vi "Send_string_to_MCU.vi"() -> (0 "STOP ALL 2":bool)   [LabVIEW 2016]
uses:
  Typedef/MCU_addresses.ctl
  Typedef/Type_of_message_to_MCU.ctl
  Typedef/Type_of_request.ctl
panel:
  in  "Ring":T1 items=["Unknown", "Neo-Pixel", "Fan Control", "Heat Control", "Display Text"]
  out "error out":errorcluster
  in  "String":string
  in  "Send To MCU":bool
  out "Byte array has been sent":u8[](array[numeric])
  out "Converted Message":string
  in  "Types of Data":T2
  in  "MCU Address to be sent":T3
  in  "EXIT":bool
  in  "STOP ALL":bool
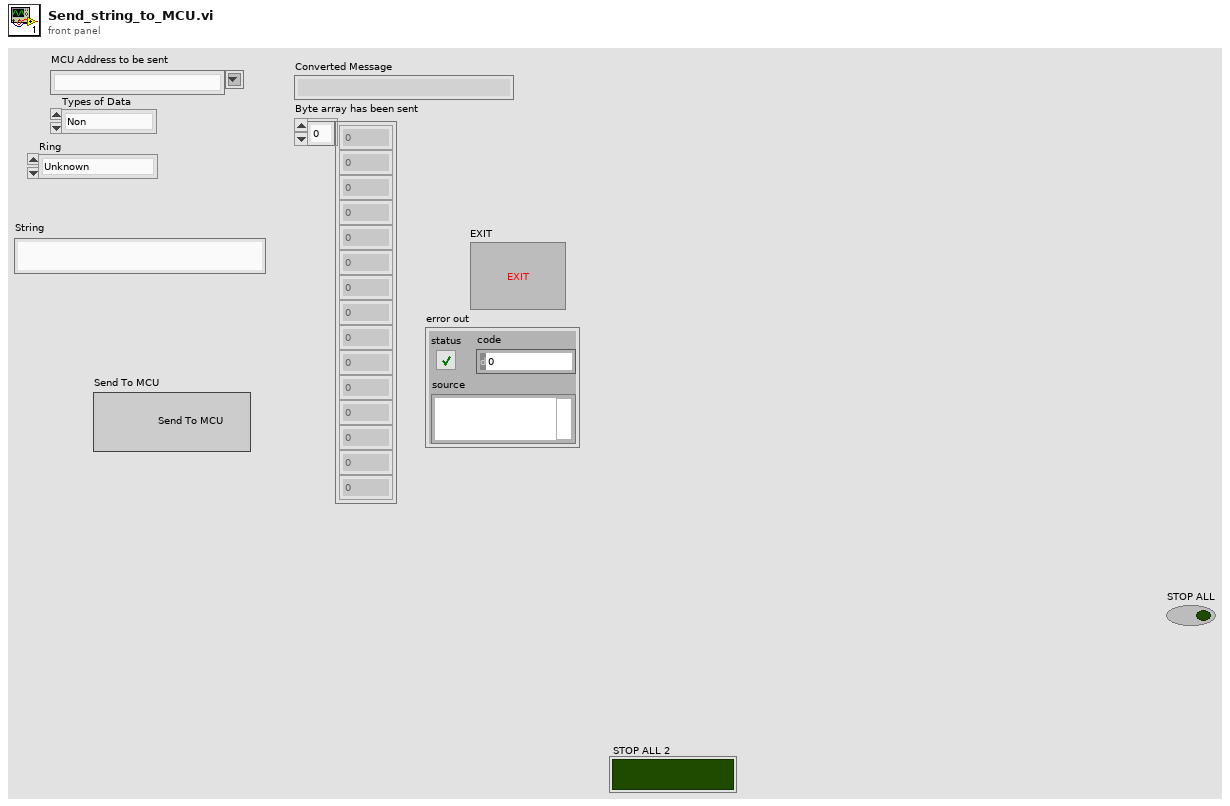
[diagram p1: front panel]
types:
  T1 = typedef "Type_of_request.ctl" = u8
  T2 = typedef "Type_of_message_to_MCU.ctl" = enum16{"Non", "Alarm", "Error", "Time and Date", "Status", "Request", "Command"}
  T3 = typedef "MCU_addresses.ctl" = string
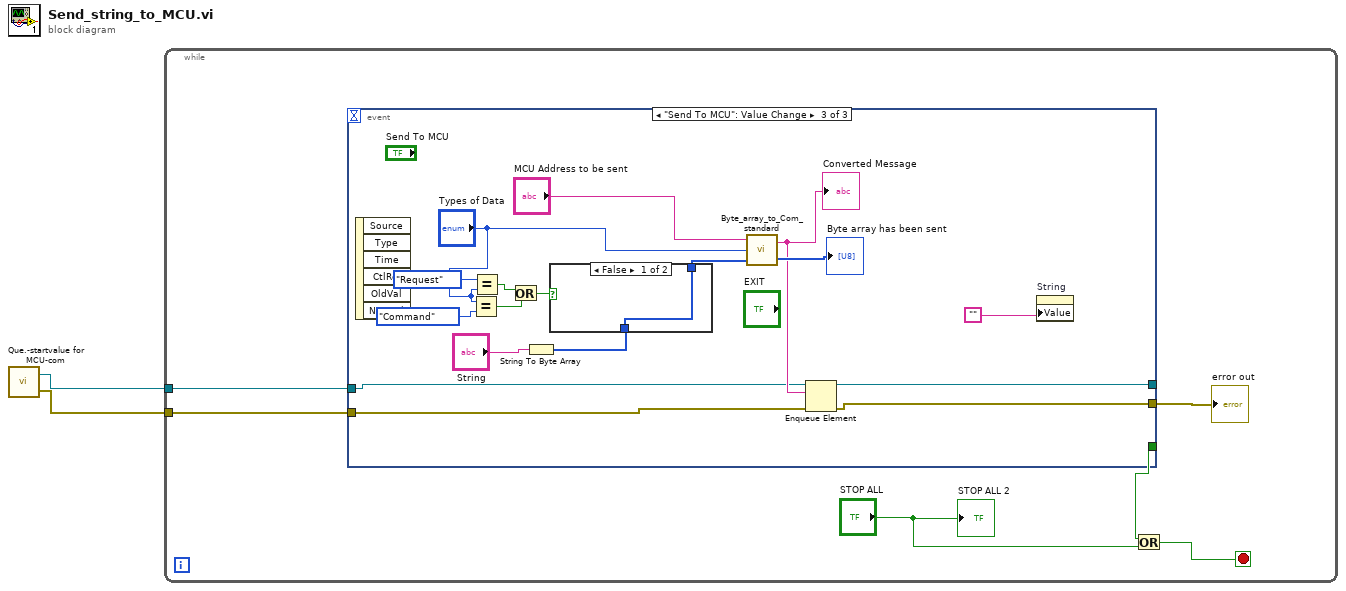
[diagram p0: block diagram]
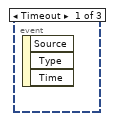
[diagram p2: hidden frame]
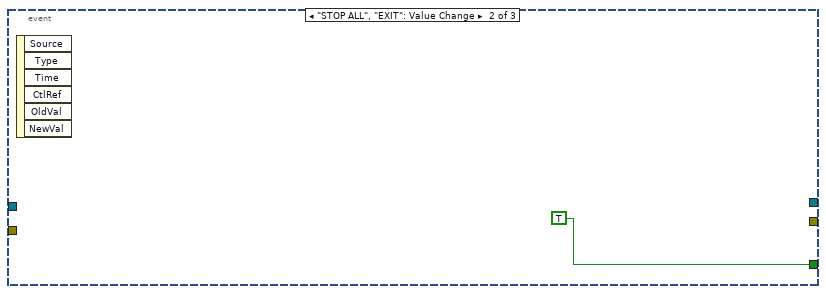
[diagram p3: hidden frame]
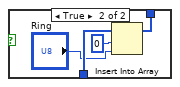
[diagram p4: hidden frame]
diagram:
  n1 = call "Que.-startvalue for MCU-com.vi"() -> ("error out"=w1:errorcluster, "queue out"=w2:refnum<queue>)  [unwired: 2 in]
  n2 = while {
    tunnel: w2 -> [w5]
    tunnel: w1 -> [w4]
    stop <- w6 stop-if-true
    n3 = event shown="[2] \"Send To MCU\": Value Change" {
      selector: _ -> [_ _ _]
      dyn-events: _ -> [_ _ _]
      timeout: _ -> [_ _ _]
      tunnel: [_ TRUE _] -> w7
      tunnel: w5 -> [_ _ w23]
      tunnel: w4 -> [_ _ w22]
      tunnel: [_ _ w19] -> _
      tunnel: [_ _ w18] -> w3
      event Timeout {
        n4 = event-data() -> ()  [unwired: 1 in, 3 out]
      }
      event "STOP ALL", "EXIT": Value Change {
        n5 = event-data() -> ()  [unwired: 1 in, 6 out]
      }
      event "Send To MCU": Value Change {
        n6 = event-data() -> ()  [unwired: 1 in, 6 out]
        n7 = Equal?(x="Types of Data", y=Type_of_message_to_MCU."Command" ("Types of Data")) -> (x = y?=w13:bool)
        n8 = Equal?(x=Type_of_message_to_MCU."Request", y="Types of Data") -> (x = y?=w14:bool)
        n9 = Or(x=w14, y=w13) -> (x .or. y?=w15:bool)
        n10 = String To Byte Array(string="String") -> (unsigned byte array=w17:u8[])
        n11 = case shown="False" w15 {
          tunnel: w17 -> [w27 w31]
          tunnel: [w27 w29] -> w16
          frame False {
          }
          frame True {
            n12 = Insert Into Array(array=w31, index=0, new element="Ring") -> (w29:u8[])
          }
        }
        n13 = call "Byte_array_to_Com_standard.vi"("Payload  Byte to be sent"=w16, "Types of Data"="Types of Data", "MCU Address to be sent"="MCU Address to be sent") -> ("Byte array has been sent"=→"Byte array has been sent":u8[], "Converted Message"=w24:string)
        "Converted Message" <- w24
        n14 = Enqueue Element(queue=w23, element=w24, error in (no error)=w22) -> (queue out=w19:refnum<queue>, error out=w18:errorcluster)  [unwired: 1 in, 1 out]
        n15 = property on="String" class="Str"("Value"="") -> ()  [unwired: 2 in, 2 out]
      }
    }
    "error out" <- w3
    n16 = Or(x=w7, y="STOP ALL") -> (x .or. y?=w6:bool)
    "STOP ALL 2" <- "STOP ALL"
  }
